vi "Get Instr Ident.vi"(8 "error in":errorcluster, 11 "Copy of PCAN in":refnum<class "PCAN.lvclass">) -> (0 "error out":errorcluster, 2 "Instr Ident":string, 3 "Copy of PCAN out":refnum<class "PCAN.lvclass">)   [LabVIEW 2024, in "PCAN.lvlib" / "PCAN.lvclass"]
uses:
  PCAN.lvclass
  PCAN.lvclass/PCAN.ctl
  Interfaces/IConfigure/IConfigure.lvclass
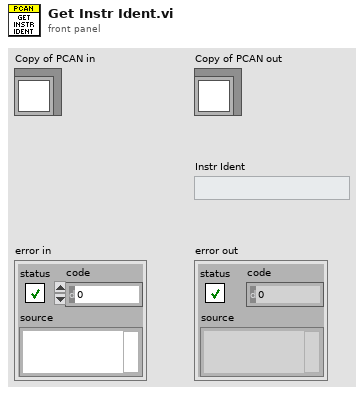
[diagram p1: front panel]
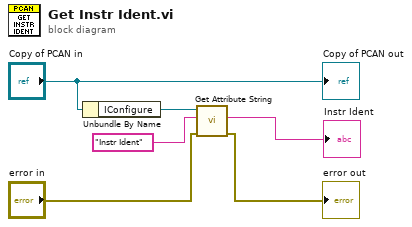
[diagram p0: block diagram]
diagram:
  n1 = Unbundle By Name("Copy of PCAN in") -> ("IConfigure"=w5:refnum<class "IConfigure.lvclass">)
  n2 = call-dynamic "Get Attribute String.vi"("error in"="error in", "Attribute"="Instr Ident", "IConfigure in"=w5) -> ("error out"=→"error out":errorcluster, "Value"=→"Instr Ident":string)  [unwired: 6 in, 1 out]
  "Copy of PCAN out" <- "Copy of PCAN in"
